vi "Update GPM Repo if needed.vi"(8 "error in (no error)":errorcluster, 11 "Repos in":refnum<class "Repo.lvclass">[](array[class])) -> (0 "error out":errorcluster, 2 "Updated?":bool, 3 "Repos out":refnum<class "Repo.lvclass">[](array[class]))   [LabVIEW 2020, in "Packages.lvlib" / "GPM.lvlib"]
uses:
  GPM.lvlib
  Repo_class/Repo.lvclass
  Repo_class/RepoType--enum.ctl
  Repo_class/Repo.lvclass/Repo.ctl
  Repo_class/Read RepoType.vi
  Repo_class/Read LastUpdated.vi
  WSsupport/WSsupport.lvlib
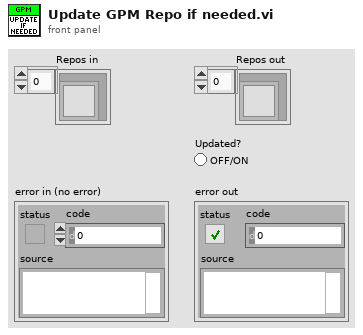
[diagram p1: front panel]
types:
  T1 = typedef "Packages.lvlib/Repo.lvclass/RepoType--enum.ctl" = enum16{"VIPM", "NIPM", "GPM"}
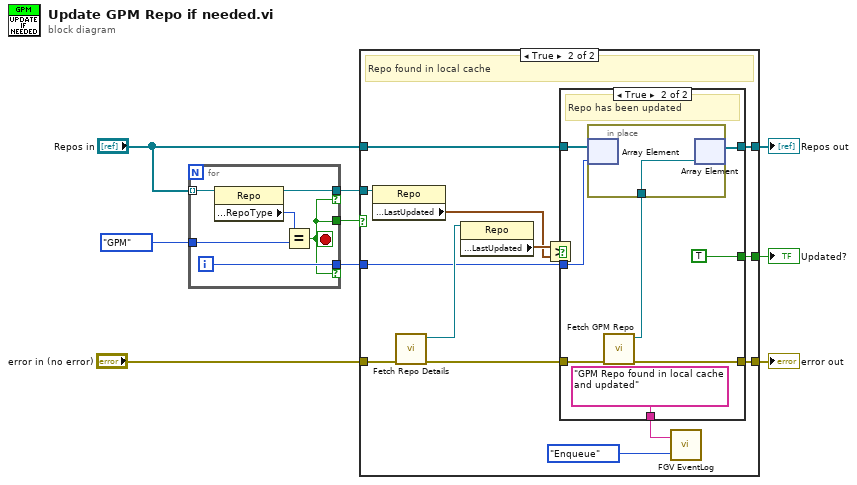
[diagram p0: block diagram]
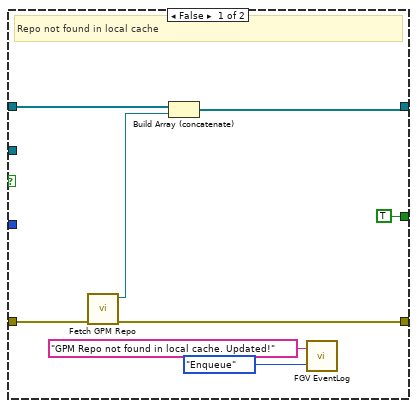
[diagram p2: hidden frame]
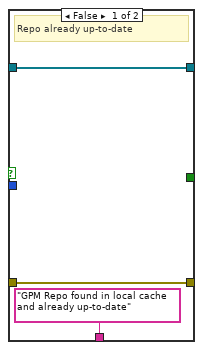
[diagram p3: hidden frame]
diagram:
  n1 = for {
    tunnel: "Repos in" -> [w15] mode=indexing
    tunnel: RepoType--enum."GPM" ("RepoType") -> [w14]
    tunnel: [w12] -> w5 if=w10
    tunnel: [w10] -> w8
    tunnel: [w11] -> w4 if=w10
    i -> [w11]
    stop <- w10 stop-if-true
    n2 = property class="Repo"(reference=w15) -> (reference out=w12:refnum<class "Repo.lvclass">, "Accessors:RepoType"=w13:T1)  [unwired: 1 in, 1 out]
    n3 = Equal?(x=w13, y=w14) -> (x = y?=w10:bool)
  }
  n4 = case shown="True" w8 {
    tunnel: "Repos in" -> [w22 w29]
    tunnel: "error in (no error)" -> [w23 w37]
    tunnel: [w20 w28] -> w3
    tunnel: [w19 w30] -> w6
    tunnel: w5 -> [_ w36]
    tunnel: w4 -> [_ w31]
    tunnel: [TRUE w26] -> w2
    frame False {
      # "Repo not found in local cache"
      n5 = call "Fetch GPM Repo.vi"("error in (no error)"=w23) -> ("error out"=w20:errorcluster, "Repo"=w21:refnum<class "Repo.lvclass">)  [unwired: 9 in]
      n6 = Build Array (concatenate)(w22, w21) -> (w19:refnum<class "Repo.lvclass">[])
      n7 = call "FGV EventLog.vi"("Action"=enum16{"Reset", "Enqueue", "Dequeue"}."Enqueue", "String to log"="GPM Repo not found in local cache. Updated!") -> ()  [unwired: 1 in, 1 out]
    }
    frame True {
      # "Repo found in local cache"
      n8 = property class="Repo"(reference=w36) -> ("Accessors:LastUpdated"=w33:timestamp)  [unwired: 1 in, 2 out]
      n9 = call "Fetch Repo Details.vi"("error in (no error)"=w37) -> ("error out"=w27:errorcluster, "Repo"=w35:refnum<class "Repo.lvclass">)  [unwired: 9 in]
      n10 = property class="Repo"(reference=w35) -> ("Accessors:LastUpdated"=w34:timestamp)  [unwired: 1 in, 2 out]
      n11 = Greater?(x=w34, y=w33) -> (0:w32:bool)
      n12 = case shown="True" w32 {
        tunnel: w31 -> [_ w45]
        tunnel: [w40 w43] -> w30
        tunnel: w29 -> [w40 w46]
        tunnel: [w39 w47] -> w28
        tunnel: w27 -> [w39 w48]
        tunnel: [_ TRUE] -> w26
        tunnel: ["GPM Repo found in local cache and already up-to-date" ("String to log") "GPM Repo found in local cache and updated" ("String to log")] -> w24
        frame False {
          # "Repo already up-to-date"
        }
        frame True {
          # "Repo has been updated"
          n13 = call "Fetch GPM Repo.vi"("error in (no error)"=w48) -> ("error out"=w47:errorcluster, "Repo"=w44:refnum<class "Repo.lvclass">)  [unwired: 9 in]
          n14 = in-place {
            in-place-border: w44 -> [w49]
            n15 = in-place-array #1(w46, w45) -> ()  [unwired: 1 out]
            n16 = in-place-array #1(w49) -> (w43:refnum<class "Repo.lvclass">[])  [unwired: 1 out]
          }
        }
      }
      n17 = call "FGV EventLog.vi"("Action"=enum16{"Reset", "Enqueue", "Dequeue"}."Enqueue", "String to log"=w24) -> ()  [unwired: 1 in, 1 out]
    }
  }
  "Repos out" <- w6
  "error out" <- w3
  "Updated?" <- w2
